vi "SVT Power Spectrum (N Ch).vi"(0 "scaled signals [EU]":waveform(dbl)[](array[waveform]), 2 "window":T8=1 items=["None"=0, "Hanning"=1, "Hamming"=2, "Blackman-Harris"=3, "Exact Blackman"=4, "Blackman"=5, "Flat Top"=6, "4 Term B-Harris "=7, "7 Term B-Harris"=8, "Low Sidelobe"=9, "Blackman Nuttall"=11, "Triangle"=30, "Bartlett-Hanning"=31, "Bohman"=32, "Parzen"=33, "Welch"=34, "Kaiser"=60, "Dolph-Chebyshev"=61, "Gaussian"=62], 4 "dB On (T)":bool=TRUE, 5 "error in (no error)":errorcluster, 7 "averaging parameters":T7={"averaging mode"=enum."No averaging", "weighting mode"=enum."Exponential", "number of averages"=10, "linear mode"=enum."One shot"}, 9 "restart averaging (F)":bool) -> (11 "averaging done":bool, 13 "averages completed":dbl, 14 "power spectra [dB EU]":cluster{"f0":dbl, "df":dbl, "magnitude":dbl[]}[](array[cluster]) {"magnitude" format="%.2p"; "df" format="%.2p"; "f0" format="%.2p"}, 15 "unit labels":string[](array[string]), 18 "spectrum info":T1[](array[typedef]) {"x-axis units" items=["Time (s)"=0, "Frequency-CB (Hz)"=1, "Frequency-CPB (Hz)"=1248, "Frequency-Arbitrary (Hz)"=2357, "Quefrency (s)"=2, "Revolutions (rev)"=3, "Order"=4, "Speed (RPM)"=11, "Speed (rad/s)"=21, "Index"=65535]; "weighting filter" items=["Linear", "A-weighting", "B-weighting", "C-weighting", "ITU-R 468-4", "Dolby", "CCITT", "C-message", "Wb", "Wc", "Wd", "We", "Wf", "Wh", "Wj", "Wk", "Wm", "AES17 20 kHz lowpass", "AES17 40 kHz lowpass", "AES17 20 kHz highpass", "AES17 40 kHz highpass"]; "dB reference [EU]" format="%.2f"; "engineering units" items=["custom..."=0, "V"=1, "A"=21, "C"=30, "pC"=31, "s"=32, "-"=29, "Pa"=2, "N"=20, "g"=3, "m/s^2"=4, "m/s"=5, "m"=6, "mm/s"=12, "mm"=13, "micron/s"=14, "micron"=15, "in/s^2"=7, "in/s"=8, "in"=9, "mil/s"=10, "mil"=11, "rad/s^2"=16, "rad/s"=17, "rad"=18, "deg/s^2"=26, "deg/s"=27, "deg"=28, "RPM"=22, "cycle/s^2"=23, "Hz"=24, "cycle"=25, "strain"=19]; "spectral info"."window" items=["None "=0, "Hanning"=1, "Hamming"=2, "Blackman-Harris"=3, "Exact Blackman"=4, "Blackman"=5, "Flat Top"=6, "4 Term B-Harris "=7, "7 Term B-Harris"=8, "Low Sidelobe"=9, "Force - Exponential"=10, "Gaussian"=62]}, 19 "error out":errorcluster)   [LabVIEW 2017]
doc: "Computes the power spectrum of <B>scaled signal [EU]</B>. You can use this polymorphic VI to analyze signals from a single channel or from N channels. The data type you wire to the <B>scaled signal [EU]</B> input determines the polymorphic instance to use."
uses:
  <vilib>/addons/_NISVFA/_Shared subVIs/Controls/svc_Window.ctl
  <vilib>/addons/_NISVFA/_Shared subVIs/Controls/svc_Spectrum Info.ctl
  <vilib>/addons/_NISVFA/_Shared subVIs/Controls/svc_X-Axis Units.ctl
  <vilib>/addons/_NISVFA/_Shared subVIs/Controls/svc_Spectrum Type.ctl
  <vilib>/addons/_NISVFA/_Shared subVIs/Controls/svc_Engineering Units Text Ring.ctl
  <vilib>/addons/_NISVFA/_Shared subVIs/Controls/svc_Weighting Filter Text Ring.ctl
  <vilib>/addons/_NISVFA/_Shared subVIs/Controls/svc_Complimentary Spectrum Units.ctl
  <vilib>/addons/_NISVFA/_Baseband FFT/SVFA Power Spectrum (N Ch).vi
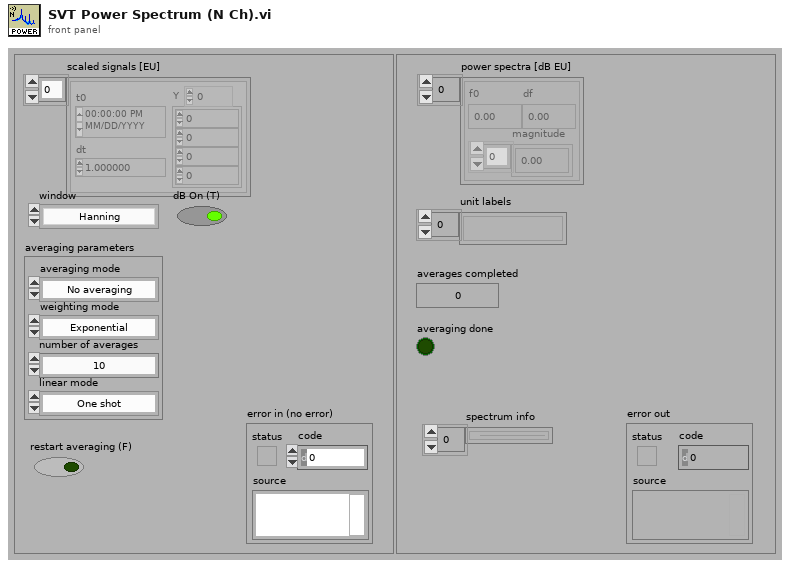
[diagram p1: front panel]
types:
  T1 = typedef "svc_Spectrum Info.ctl" = cluster{"channel name":string, "description":string, "x-axis units":T2, "spectral info":cluster{"spectrum type":T3, "linear/dB":enum16{"linear", "dB"}, "window":u16, "window size":i32, "FFT size":i32}, "engineering units":T4, "custom label":string, "dB reference [EU]":dbl, "peak units":enum16{"rms", "peak", "peak-peak"}, "weighting filter":T5, "spectral density?":bool, "unit label":string, "spectrum skewed?":bool, "complimentary spectrum units":T6}
  T2 = typedef "svc_X-Axis Units.ctl" = u16
  T3 = typedef "svc_Spectrum Type.ctl" = enum16{"FFT Spectrum [complex]", "Amplitude [Magnitude]", "Power [Magnitude^2]", "Cross Spectrum [complex]", "Frequency Response [Complex]"}
  T4 = typedef "svc_Engineering Units Text Ring.ctl" = u16
  T5 = typedef "svc_Weighting Filter Text Ring.ctl" = u16
  T6 = typedef "svc_Complimentary Spectrum Units.ctl" = enum16{"none", "radians", "degrees", "cycles", "imaginary"}
  T7 = cluster{"averaging mode":enum16{"No averaging", "Vector averaging", "RMS averaging", "Peak hold"}, "weighting mode":enum16{"Linear", "Exponential"}, "number of averages":u32, "linear mode":enum16{"One shot", "Auto restart"}}
  T8 = typedef "svc_Window.ctl" = u32
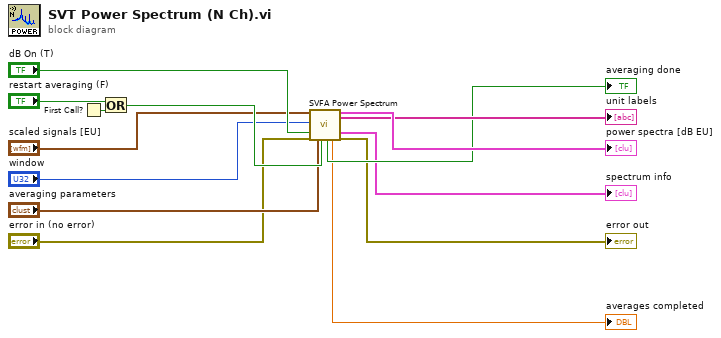
[diagram p0: block diagram]
diagram:
  n1 = First Call?() -> (First Call?: T/F=w14:bool)
  n2 = Or(x="restart averaging (F)", y=w14) -> (x .or. y?=w11:bool)
  n3 = call-poly <vilib>:"SVFA Power Spectrum.vi"("scaled signals [EU]"="scaled signals [EU]", "window"="window", "dB On (T)"="dB On (T)", "error in (no error)"="error in (no error)", "averaging parameters"="averaging parameters", "restart averaging (F)"=w11) -> ("averaging done"=→"averaging done":bool, "averages completed"=→"averages completed":dbl, "power spectra [dB EU]"=→"power spectra [dB EU]":cluster{"f0":dbl, "df":dbl, "magnitude":dbl[]}[], "unit labels"=→"unit labels":string[], "spectrum info"=→"spectrum info":T1[], "error out"=→"error out":errorcluster)  [unwired: 8 in]
